vi "dll_tester.vi"() -> ()   [LabVIEW 2020]
uses:
  JLinkARM.lvlib
panel:
  out "error out":errorcluster caption="错误输出"
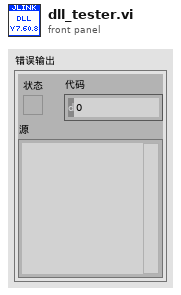
[diagram p1: front panel]
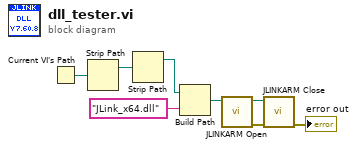
[diagram p0: block diagram]
diagram:
  n1 = Current VI's Path() -> (path=w3:path)
  n2 = Strip Path(path=w3) -> (stripped path=w2:path)  [unwired: 1 out]
  n3 = Strip Path(path=w2) -> (stripped path=w1:path)  [unwired: 1 out]
  n4 = Build Path(base path=w1, name or relative path="JLink_x64.dll") -> (appended path=w6:path)
  n5 = call <userlib>:"JLINKARM Open.vi"("path in"=w6) -> ("error out"=w7:errorcluster, "path out"=w8:path)  [unwired: 9 in]
  n6 = call <userlib>:"JLINKARM Close.vi"("error in (no error)"=w7, "path in"=w8) -> ("error out"=→"error out":errorcluster)  [unwired: 8 in, 1 out]
